vi "Debouncer_New.vi"(8 "CurrentTIme":dbl=-1.0, 10 "DebounceType":T1, 11 "DebounceTime":dbl) -> (0 "CurrentTIme Out":dbl=-1.0, 3 "Debouncer":T2 {"PrevTimeSeconds" format="%13.6p"; "DebounceTimeSeconds" format="%13.6p"})   [LabVIEW 2019, in "Trajectory_Library.lvlib"]
doc: "A simple debounce filter for boolean streams. Requires that the boolean change value from baseline for a specified period of time before the filtered value changes.\n\nCreates a new Debouncer.\n\nInputs:\n - DebounceTime -- The number of seconds the value must change from baseline for the filtered value to change.\n - DebounceType -- Which type of state change the debouncing will be performed on. (Optional: Default: Rising)\n - CurrentTime -- Current system running time. (Optional - Default: Read system time.)\n\nOutput:\n - Debouncer -- Initialized data cluster for debouncer."
uses:
  Trajectory_Library.lvlib
  Enum/DEBOUNCER_TYPE_ENUM.ctl
  TypeDef/DEBOUNCER.ctl
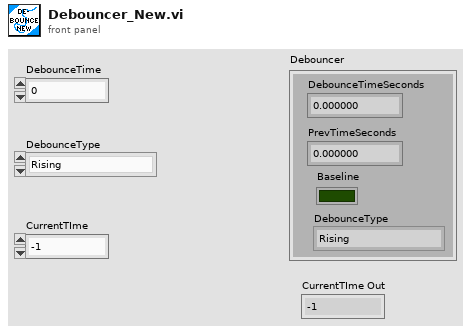
[diagram p1: front panel]
types:
  T1 = typedef "Trajectory_Library.lvlib/DEBOUNCER_TYPE_ENUM.ctl" = enum16{"Rising", "Falling", "Both"}
  T2 = typedef "Trajectory_Library.lvlib/DEBOUNCER.ctl" = cluster{"DebounceTimeSeconds":dbl, "PrevTimeSeconds":dbl, "Baseline":bool, "DebounceType":T1}
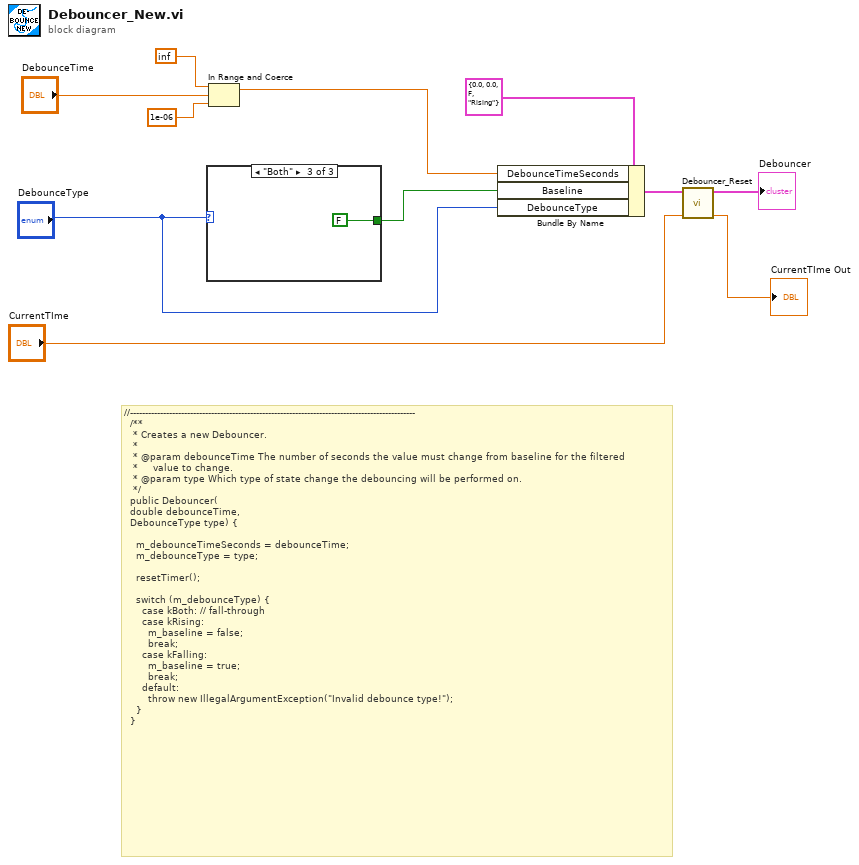
[diagram p0: block diagram]
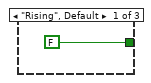
[diagram p2: hidden frame]
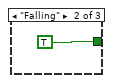
[diagram p3: hidden frame]
diagram:
  # "//-----------------------------------------------------------------------------------------------\n  /**\n   * Creates a new Debouncer.\n   *\n   * @param debounceTime The number of seconds the value must change from baseline for the filtered\n   *     value to change.\n   * @param type Which type of state change the debouncing will be performed on.\n   */\n  public Debouncer(\n\t\tdouble debounceTime, \n\t\tDebounceType type) {\n\n    m_debounceTimeSeconds = debounceTime;\n    m_debounceType = type;\n\n    resetTimer();\n\n    switch (m_debounceType) {\n      case kBoth: // fall-through\n      case kRising:\n        m_baseline = false;\n        break;\n      case kFalling:\n        m_baseline = true;\n        break;\n      default:\n        throw new IllegalArgumentException(\"Invalid debounce type!\");\n    }\n  }"
  n1 = case shown="\"Both\"" "DebounceType" {
    tunnel: [FALSE TRUE FALSE] -> w10
    frame "Rising", Default {
    }
    frame "Falling" {
    }
    frame "Both" {
    }
  }
  n2 = In Range and Coerce(upper limit=inf, x="DebounceTime", lower limit=1e-06) -> (coerced(x)=w5:dbl)  [unwired: 1 out]
  n3 = Bundle By Name(cluster=T2 {"DebounceTimeSeconds"=0.0, "PrevTimeSeconds"=0.0, "Baseline"=FALSE, "DebounceType"=enum."Rising"} ("Debouncer 2"), "DebounceTimeSeconds"=w5, "Baseline"=w10, "DebounceType"="DebounceType") -> (w4:T2)
  n4 = call "Debouncer_Reset.vi"("CurrentTIme"="CurrentTIme", "Debouncer In"=w4) -> ("CurrentTIme Out"=→"CurrentTIme Out":dbl, "Debouncer Out"=→"Debouncer":T2)  [unwired: 8 in]
